vi "Risposta Server.vi"() -> ()   [LabVIEW 2022 SP3]
panel:
  in  "Scelta server":enum16{"Server 01", "Server 02"}(ring)
  in  "String Array":string[](array[string])
  out "Risposta Server":string[](array[string])
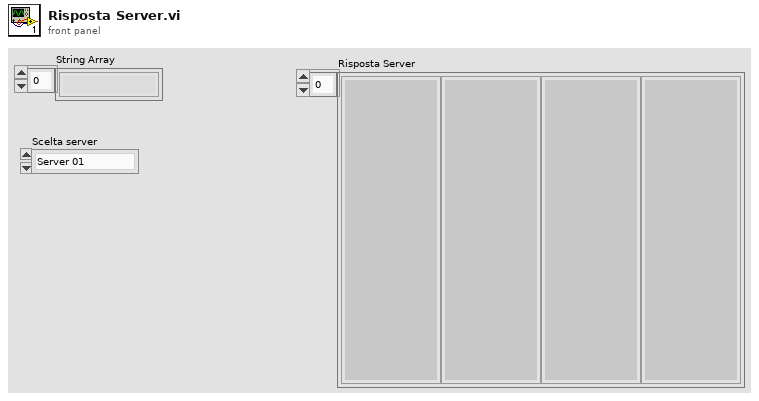
[diagram p1: front panel]
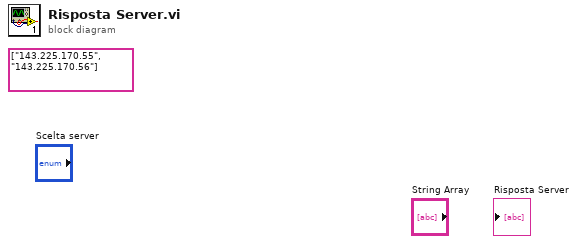
[diagram p0: block diagram]
diagram:
  (unwired) string[] ["143.225.170.55", "143.225.170.56"]
